vi "read refnum - polymorphic.vi"   [LabVIEW 2024, in "controls manager.lvlib"]
uses:
  controls manager.lvlib
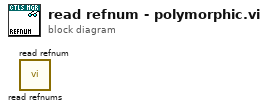
[diagram p0: block diagram]
diagram:
  n1 = call "read refnums.vi"() -> ()  [unwired: 10 in, 2 out]
  n2 = call "read refnum.vi"() -> ()  [unwired: 10 in, 2 out]
